vi "Interface Prototype.vi"() -> ()   [LabVIEW 2015, in "niInstr Streaming v1 FPGA.lvlib"]
uses:
  <instrlib>/_niInstr/Streaming/v1/FPGA/niInstr Streaming v1 FPGA.lvlib
  <instrlib>/_niInstr/Streaming/v1/Common/Stream State.ctl
  <instrlib>/_niInstr/Streaming/v1/Common/niInstr Streaming v1 Common.lvlib
panel:
  out "stream.state 15":T1
  out "stream.state 14":T1
  out "stream.state 13":T1
  out "stream.state 12":T1
  out "stream.state 11":T1
  out "stream.state 10":T1
  out "stream.state 9":T1
  out "stream.state 8":T1
  out "stream.state 7":T1
  out "stream.state 6":T1
  out "stream.state 5":T1
  out "stream.state 4":T1
  out "stream.state 3":T1
  out "stream.state 2":T1
  out "stream.state 1":T1
  out "stream.state 0":T1
  out "stream.min samples ready 15":u32
  out "stream.min samples ready 14":u32
  out "stream.min samples ready 13":u32
  out "stream.min samples ready 12":u32
  out "stream.min samples ready 11":u32
  out "stream.min samples ready 10":u32
  out "stream.min samples ready 9":u32
  out "stream.min samples ready 8":u32
  out "stream.min samples ready 7":u32
  out "stream.min samples ready 6":u32
  out "stream.min samples ready 5":u32
  out "stream.min samples ready 4":u32
  out "stream.min samples ready 3":u32
  out "stream.min samples ready 2":u32
  out "stream.min samples ready 1":u32
  out "stream.min samples ready 0":u32
  out "stream.max samples ready 15":u32
  out "stream.max samples ready 14":u32
  out "stream.max samples ready 13":u32
  out "stream.max samples ready 12":u32
  out "stream.max samples ready 11":u32
  out "stream.max samples ready 10":u32
  out "stream.max samples ready 9":u32
  out "stream.max samples ready 8":u32
  out "stream.max samples ready 7":u32
  out "stream.max samples ready 6":u32
  out "stream.max samples ready 5":u32
  out "stream.max samples ready 4":u32
  out "stream.max samples ready 3":u32
  out "stream.max samples ready 2":u32
  out "stream.max samples ready 1":u32
  out "stream.max samples ready 0":u32
  in  "stream.minimum elements to start 15":u32
  in  "stream.minimum elements to start 14":u32
  in  "stream.minimum elements to start 13":u32
  in  "stream.minimum elements to start 12":u32
  in  "stream.minimum elements to start 11":u32
  in  "stream.minimum elements to start 10":u32
  in  "stream.minimum elements to start 9":u32
  in  "stream.minimum elements to start 8":u32
  in  "stream.minimum elements to start 7":u32
  in  "stream.minimum elements to start 6":u32
  in  "stream.minimum elements to start 5":u32
  in  "stream.minimum elements to start 4":u32
  in  "stream.minimum elements to start 3":u32
  in  "stream.minimum elements to start 2":u32
  in  "stream.minimum elements to start 1":u32
  in  "stream.minimum elements to start 0":u32
  in  "stream.reset health monitor 15":bool
  in  "stream.reset health monitor 14":bool
  in  "stream.reset health monitor 13":bool
  in  "stream.reset health monitor 12":bool
  in  "stream.reset health monitor 11":bool
  in  "stream.reset health monitor 10":bool
  in  "stream.reset health monitor 9":bool
  in  "stream.reset health monitor 8":bool
  in  "stream.reset health monitor 7":bool
  in  "stream.reset health monitor 6":bool
  in  "stream.reset health monitor 5":bool
  in  "stream.reset health monitor 4":bool
  in  "stream.reset health monitor 3":bool
  in  "stream.reset health monitor 2":bool
  in  "stream.reset health monitor 1":bool
  in  "stream.reset health monitor 0":bool
  out "stream.num samples ready 15":u32
  out "stream.num samples ready 14":u32
  out "stream.num samples ready 13":u32
  out "stream.num samples ready 12":u32
  out "stream.num samples ready 11":u32
  out "stream.num samples ready 10":u32
  out "stream.num samples ready 9":u32
  out "stream.num samples ready 8":u32
  out "stream.num samples ready 7":u32
  out "stream.num samples ready 6":u32
  out "stream.num samples ready 5":u32
  out "stream.num samples ready 4":u32
  out "stream.num samples ready 3":u32
  out "stream.num samples ready 2":u32
  out "stream.num samples ready 1":u32
  out "stream.num samples ready 0":u32
  out "stream.metadata 15":u64
  out "stream.metadata 14":u64
  out "stream.metadata 13":u64
  out "stream.metadata 12":u64
  out "stream.metadata 11":u64
  out "stream.metadata 10":u64
  out "stream.metadata 9":u64
  out "stream.metadata 8":u64
  out "stream.metadata 7":u64
  out "stream.metadata 6":u64
  out "stream.metadata 5":u64
  out "stream.metadata 4":u64
  out "stream.metadata 3":u64
  out "stream.metadata 2":u64
  out "stream.metadata 1":u64
  out "stream.metadata 0":u64
  out "stream.samples transferred 15":u64
  out "stream.samples transferred 14":u64
  out "stream.samples transferred 13":u64
  out "stream.samples transferred 12":u64
  out "stream.samples transferred 11":u64
  out "stream.samples transferred 10":u64
  out "stream.samples transferred 9":u64
  out "stream.samples transferred 8":u64
  out "stream.samples transferred 7":u64
  out "stream.samples transferred 6":u64
  out "stream.samples transferred 5":u64
  out "stream.samples transferred 4":u64
  out "stream.samples transferred 3":u64
  out "stream.samples transferred 2":u64
  out "stream.samples transferred 1":u64
  out "stream.samples transferred 0":u64
  in  "stream.num samples 15":u64
  in  "stream.num samples 14":u64
  in  "stream.num samples 13":u64
  in  "stream.num samples 12":u64
  in  "stream.num samples 11":u64
  in  "stream.num samples 10":u64
  in  "stream.num samples 9":u64
  in  "stream.num samples 8":u64
  in  "stream.num samples 7":u64
  in  "stream.num samples 6":u64
  in  "stream.num samples 5":u64
  in  "stream.num samples 4":u64
  in  "stream.num samples 3":u64
  in  "stream.num samples 2":u64
  in  "stream.num samples 1":u64
  in  "stream.num samples 0":u64
  in  "stream.request state 15":T1
  in  "stream.request state 14":T1
  in  "stream.request state 13":T1
  in  "stream.request state 12":T1
  in  "stream.request state 11":T1
  in  "stream.request state 10":T1
  in  "stream.request state 9":T1
  in  "stream.request state 8":T1
  in  "stream.request state 7":T1
  in  "stream.request state 6":T1
  in  "stream.request state 5":T1
  in  "stream.request state 4":T1
  in  "stream.request state 3":T1
  in  "stream.request state 2":T1
  in  "stream.request state 1":T1
  in  "stream.request state 0":T1
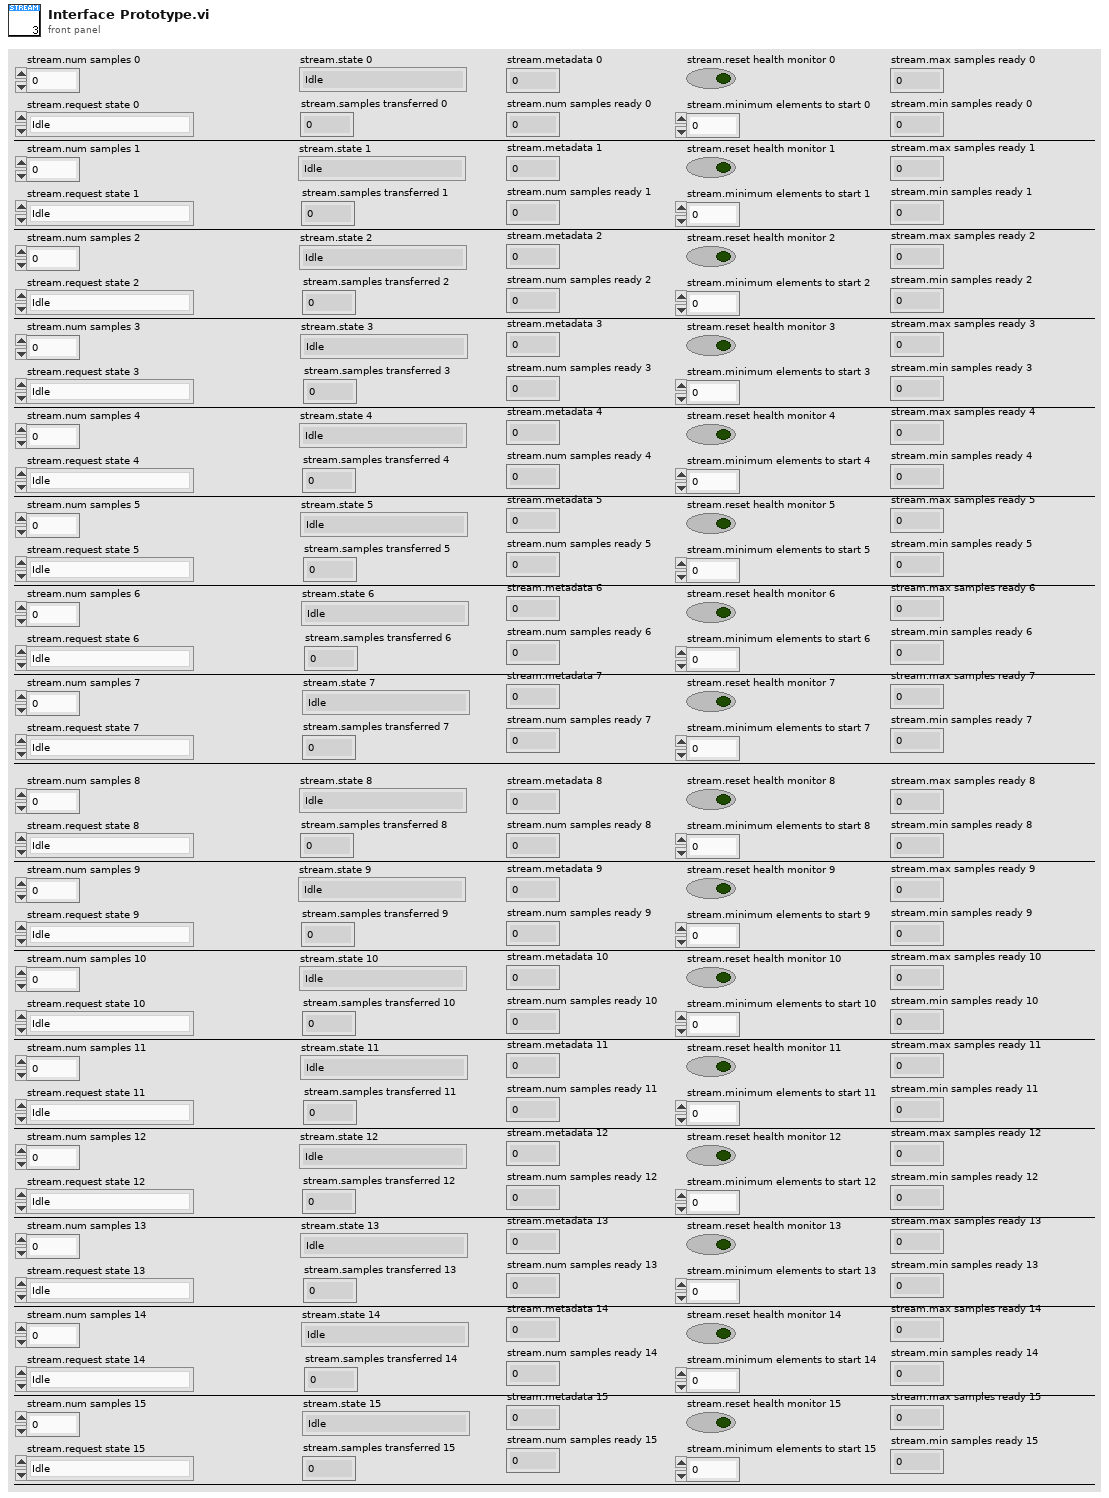
[diagram p1: front panel]
types:
  T1 = typedef "niInstr Streaming v1 Common.lvlib/Stream State.ctl" = enum8{"Idle", "Finite Transfer", "Continuous", "Done", "Error", "Not Ready", "Cancel"}
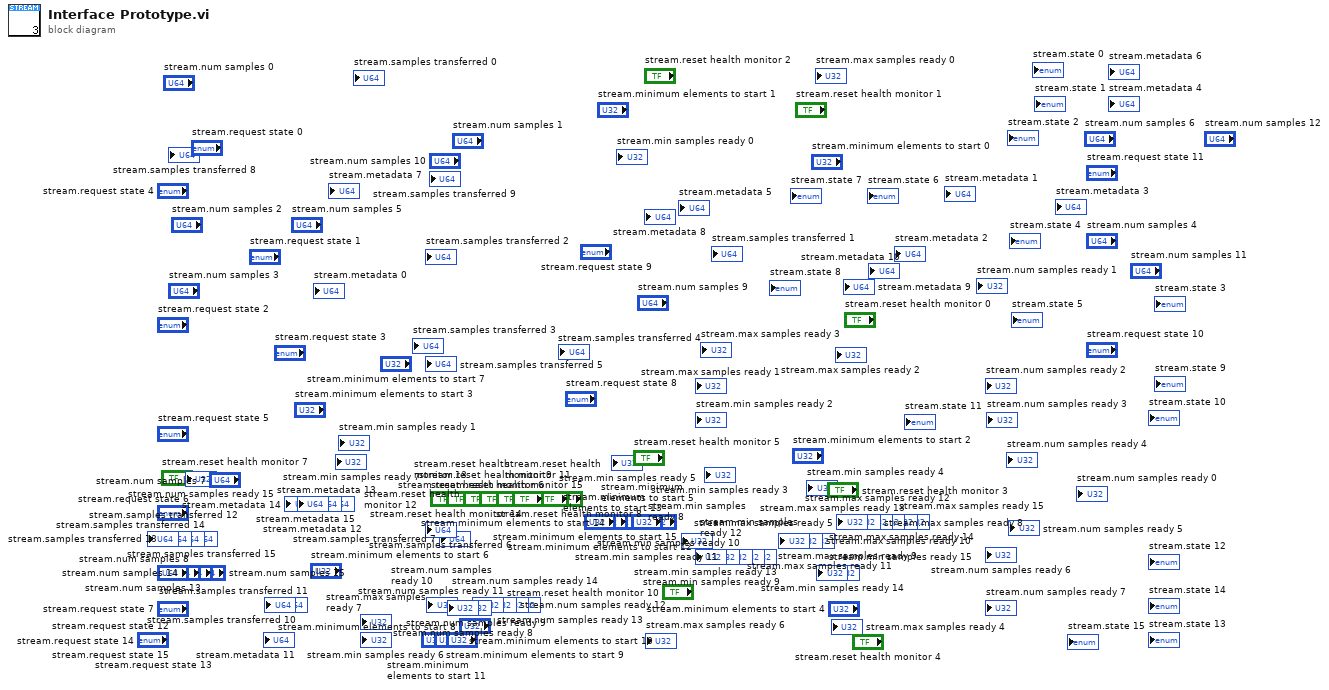
[diagram p0: block diagram]
diagram:
